vi "zmq_getsocketopt_int64.vi"(3 "error in":errorcluster, 4 "option":T1, 5 "socket in":refnum<class "Socket.lvclass">) -> (0 "error out":errorcluster, 1 "value":i64, 2 "socket out":refnum<class "Socket.lvclass">)   [LabVIEW 2025, in "ZeroMQ.lvlib" / "Socket.lvclass"]
doc: "Query the value of <b>option</b> for the given <b>socket</b>.\n\nYou are responsible for selecting the correct polymorphic instance for the option you wish to query. Valid options of type int64 are: ZMQ_AFFINITY, ZMQ_MAXMSGSIZE\n\nFurther API documentation: http://api.zeromq.org/3-2:zmq-getsockopt"
uses:
  Socket.lvclass
  Socket.lvclass/Socket.ctl
  ZeroMQ.lvlib
  socket_options.ctl
panel:
  # "ØMQ"
  # "labview"
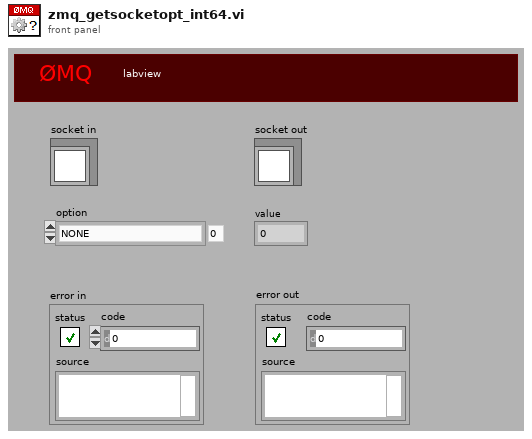
[diagram p1: front panel]
types:
  T1 = typedef "ZeroMQ.lvlib/socket_options.ctl" = enum8{"NONE", "ZMQ_HWM", "<2>", "ZMQ_SWAP", "ZMQ_AFFINITY", "ZMQ_ROUTING_ID", "ZMQ_SUBSCRIBE", "ZMQ_UNSUBSCRIBE", "ZMQ_RATE", "ZMQ_RECOVERY_IVL", "ZMQ_MCAST_LOOP", "ZMQ_SNDBUF", "ZMQ_RCVBUF", "ZMQ_RCVMORE", "ZMQ_FD", "ZMQ_EVENTS", "ZMQ_TYPE", "ZMQ_LINGER", "ZMQ_RECONNECT_IVL", "ZMQ_BACKLOG", "ZMQ_RECOVERY_IVL_MSEC", "ZMQ_RECONNECT_IVL_MAX", "ZMQ_MAXMSGSIZE", "ZMQ_SNDHWM", "ZMQ_RCVHWM", "ZMQ_MULTICAST_HOPS", "<26>", "ZMQ_RCVTIMEO", "ZMQ_SNDTIMEO", "<29>", "<30>", "ZMQ_IPV4ONLY", "ZMQ_LAST_ENDPOINT", "ZMQ_ROUTER_MANDATORY", "ZMQ_TCP_KEEPALIVE", "ZMQ_TCP_KEEPALIVE_CNT", "ZMQ_TCP_KEEPALIVE_IDLE", "ZMQ_TCP_KEEPALIVE_INTVL", "ZMQ_TCP_ACCEPT_FILTER", "ZMQ_IMMEDIATE", "ZMQ_XPUB_VERBOSE", "ZMQ_ROUTER_RAW", "ZMQ_IPV6", "ZMQ_MECHANISM", "ZMQ_PLAIN_SERVER", "ZMQ_PLAIN_USERNAME", "ZMQ_PLAIN_PASSWORD", "ZMQ_CURVE_SERVER", "ZMQ_CURVE_PUBLICKEY", "ZMQ_CURVE_SECRETKEY", "ZMQ_CURVE_SERVERKEY", "ZMQ_PROBE_ROUTER", "ZMQ_REQ_CORRELATE", "ZMQ_REQ_RELAXED", "ZMQ_CONFLATE", "ZMQ_ZAP_DOMAIN", "ZMQ_ROUTER_HANDOVER", "ZMQ_TOS", "ZMQ_IPC_FILTER_PID", "ZMQ_IPC_FILTER_UID", "ZMQ_IPC_FILTER_GID", "ZMQ_CONNECT_ROUTING_ID", "ZMQ_GSSAPI_SERVER", "ZMQ_GSSAPI_PRINCIPAL", "ZMQ_GSSAPI_SERVICE_PRINCIPAL", "ZMQ_GSSAPI_PLAINTEXT", "ZMQ_HANDSHAKE_IVL", "<67>", "ZMQ_SOCKS_PROXY", "ZMQ_XPUB_NODROP", "ZMQ_BLOCKY", "ZMQ_XPUB_MANUAL", "ZMQ_XPUB_WELCOME_MSG", "ZMQ_STREAM_NOTIFY", "ZMQ_INVERT_MATCHING", "ZMQ_HEARTBEAT_IVL", "ZMQ_HEARTBEAT_TTL", "ZMQ_HEARTBEAT_TIMEOUT", "ZMQ_XPUB_VERBOSER", "ZMQ_CONNECT_TIMEOUT", "ZMQ_TCP_MAXRT", "ZMQ_THREAD_SAFE", "<82>", "<83>", "ZMQ_MULTICAST_MAXTPDU", "ZMQ_VMCI_BUFFER_SIZE", "ZMQ_VMCI_BUFFER_MIN_SIZE", "ZMQ_VMCI_BUFFER_MAX_SIZE", "ZMQ_VMCI_CONNECT_TIMEOUT", "ZMQ_USE_FD", "ZMQ_GSSAPI_PRINCIPAL_NAMETYPE", "ZMQ_GSSAPI_SERVICE_PRINCIPAL_NAMETYPE", "ZMQ_BINDTODEVICE", "ZMQ_ZAP_ENFORCE_DOMAIN", "ZMQ_LOOPBACK_FASTPATH", "ZMQ_METADATA", "ZMQ_MULTICAST_LOOP", "ZMQ_ROUTER_NOTIFY"}
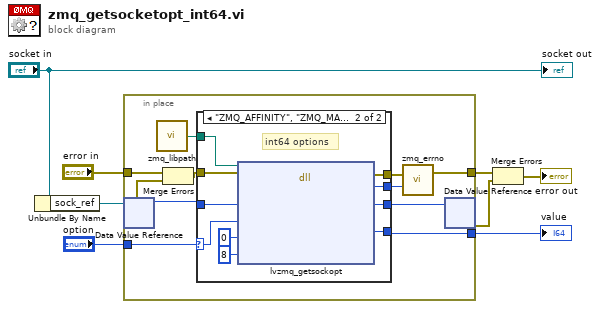
[diagram p0: block diagram]
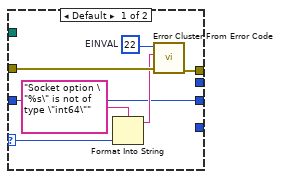
[diagram p2: hidden frame]
diagram:
  n1 = Unbundle By Name("socket in") -> ("sock_ref"=w3:refnum<data-value>)
  n2 = in-place {
    in-place-border: [w17] -> w8
    in-place-border: "error in" -> [w16]
    in-place-border: "option" -> [w15]
    in-place-border: [w14] -> w5
    n3 = in-place-dvr #1(w3) -> (w13:u64, w9:errorcluster)
    n4 = call "zmq_libpath.vi"() -> ("path"=w11:path)
    n5 = Merge Errors(w16, w9) -> (w10:errorcluster)
    n6 = case shown="\"ZMQ_AFFINITY\", \"ZMQ_MAXMSGSIZE\", \"ZMQ_VMCI_BUFFER_SIZE\"..\"ZMQ_VMCI_BUFFER_MAX_SIZE\"" w15 {
      selector: w15 -> [w23 w34]
      tunnel: [w26 w36] -> w19
      tunnel: [_ w35] -> w18
      tunnel: w10 -> [w24 w32]
      tunnel: [_ w30] -> w14
      tunnel: w13 -> [w20 w29]
      tunnel: [w20 w28] -> w12
      tunnel: w11 -> [_ w27]
      frame Default {
        w25 = 22  # EINVAL
        n7 = Format Into String(format string="Socket option \"%s\" is not of type \"int64\"", w23) -> (resulting string=w21:string)  [unwired: 2 in, 1 out]
        n8 = call <vilib>:"Error Cluster From Error Code.vi"("error in (no error)"=w24, "error message (\"\")"=w21, "error code (0)"=w25) -> ("error out"=w26:errorcluster)  [unwired: 6 in]
      }
      frame "ZMQ_AFFINITY", "ZMQ_MAXMSGSIZE", "ZMQ_VMCI_BUFFER_SIZE".."ZMQ_VMCI_BUFFER_MAX_SIZE" {
        # "int64 options"
        n9 = dll-call lib="?" fn="lvzmq_getsockopt"(path in=w27, error in=w32, "socket"=w29, "option"=w34, "data"=i64 0, "len"=u32 8) -> (error out=w36:errorcluster, "return type"=w35:i32, "socket"=w28:u64, "data"=w30:i64)  [unwired: 3 in, 1 out]
      }
    }
    n10 = call "zmq_errno.vi"("retval"=w18, "error in"=w19) -> ("error out"=w17:errorcluster)  [unwired: 1 out]
    n11 = in-place-dvr #1(w12) -> (w1:errorcluster)  [unwired: 1 out]
  }
  "value" <- w5
  n12 = Merge Errors(w8, w1) -> (→"error out":errorcluster)
  "socket out" <- "socket in"
